vi "SerialParseLines.vi"(10 "Accum In":string, 11 "Serial In":string) -> (1 "New Line Flag":bool, 2 "Line Out":string, 3 "Accum Out":string)   [LabVIEW 2015]
uses:
  <vilib>/regexp/Match Regular Expression.xnode
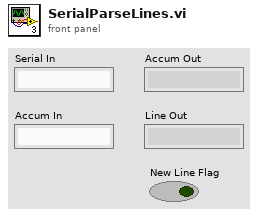
[diagram p1: front panel]
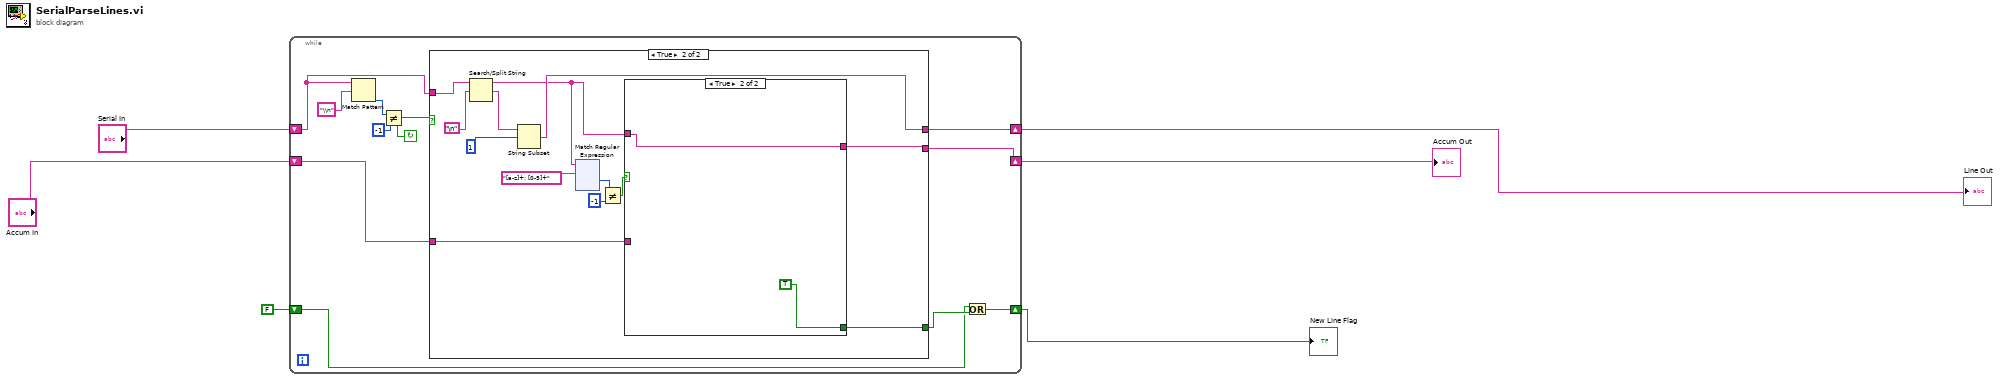
[diagram p0: block diagram]
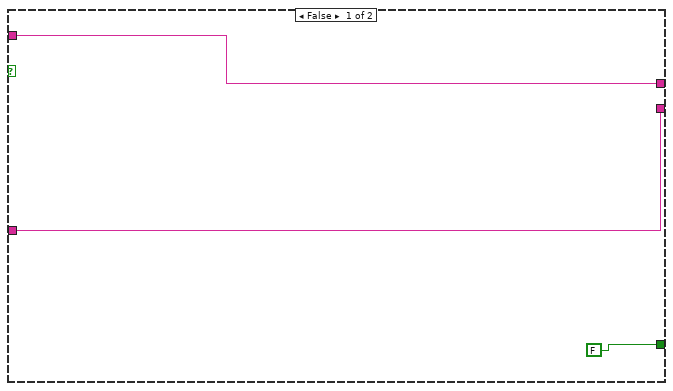
[diagram p2: hidden frame]
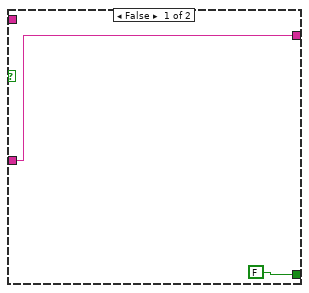
[diagram p3: hidden frame]
diagram:
  n1 = while {
    shift-right: [w14] -> w2
    shift-left: "Serial In" -> [w12]
    shift-right: [w10] -> w4
    shift-left: "Accum In" -> [w11]
    shift-right: [w7] -> w6
    shift-left: FALSE -> [w8]
    stop <- w15 continue-if-true
    n2 = Match Pattern(string=w12, regular expression="\\n") -> (offset past match=w17:i32)  [unwired: 1 in, 3 out]
    n3 = Not Equal?(x=w17, y=-1) -> (x != y?=w15:bool)
    n4 = case shown="True" w15 {
      tunnel: [w20 w31] -> w14
      tunnel: w12 -> [w20 w30]
      tunnel: w11 -> [w19 w23]
      tunnel: [w19 w22] -> w10
      tunnel: [FALSE w21] -> w9
      frame False {
      }
      frame True {
        n5 = Search/Split String(string=w30, search string/char (-)="\n") -> (substring before match=w24:string, match + rest of string=w33:string)  [unwired: 1 in, 1 out]
        n6 = String Subset(string=w33, offset (0)=1) -> (substring=w31:string)  [unwired: 1 in]
        n7 = xnode "Match Regular Expression"("input string"=w24, "regular expression"="[a-z]+: [0-9]+") -> ("offset past match"=w26:i32)  [unwired: 4 in, 4 out]
        n8 = Not Equal?(x=w26, y=-1) -> (x != y?=w27:bool)
        n9 = case shown="True" w27 {
          tunnel: w24 -> [_ w37]
          tunnel: w23 -> [w35 _]
          tunnel: [w35 w37] -> w22
          tunnel: [FALSE TRUE] -> w21
          frame False {
          }
          frame True {
          }
        }
      }
    }
    n10 = Or(x=w8, y=w9) -> (x .or. y?=w7:bool)
  }
  "New Line Flag" <- w6
  "Accum Out" <- w4
  "Line Out" <- w2
